vi "FLOW-RATE_read_flow_rate.vi"(4 "error in":errorcluster, 5 "Data t i-1":cluster{"time (s)":dbl, "volume (µl)":dbl}, 6 "FRP out":T1, 7 "Reset":bool) -> (0 "error out":errorcluster, 1 "Data t i":cluster{"time (s)":dbl, "volume (µl)":dbl}, 2 "FR (µl/min)":dbl, 3 "volume (µl)":dbl)   [LabVIEW 2015]
uses:
  <userlib>/Fluigent/Fluigent FRP/FluigentFRP.llb/_frpEnum.ctl
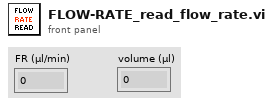
[diagram p1: front panel]
types:
  T1 = typedef "_frpRefNum" = refnum<k1>
  T2 = enum16{"Always On", "Always Off", "Off While Running"}
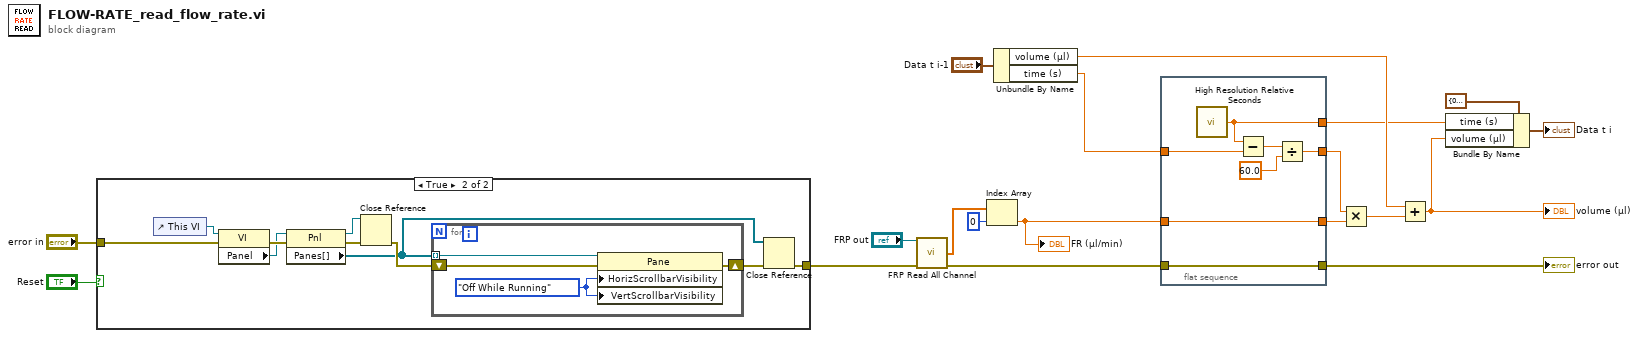
[diagram p0: block diagram]
diagram:
  n1 = case shown="True" "Reset" {
    tunnel: "error in" -> [w20 w22]
    tunnel: [w20 w21] -> w14
    frame False {
    }
    frame True {
      n2 = control-ref of="This VI"() -> (w23:refnum<vi>)
      n3 = property class="VI"(reference=w23, error in=w22) -> (error out=w25:errorcluster, "Panel"=w24:refnum<vi>)  [unwired: 1 out]
      n4 = property class="Pnl"(reference=w24, error in=w25) -> (reference out=w26:refnum<vi>, error out=w27:errorcluster, "Panes[]"=w29:refnum<vi>[])
      n5 = Close Reference(reference=w26, error in (no error)=w27) -> (error out=w30:errorcluster)
      n6 = for {
        tunnel: w29 -> [w34] mode=indexing
        shift-right: [w32] -> w28
        shift-left: w30 -> [w31]
        w33 = T2."Off While Running" ("Horizontal Scrollbar Visibility")
        n7 = property class="Pane"(reference=w34, error in=w31, "HorizScrollbarVisibility"=w33, "VertScrollbarVisibility"=w33) -> (error out=w32:errorcluster)  [unwired: 1 out]
      }
      n8 = Close Reference(reference=w29, error in (no error)=w28) -> (error out=w21:errorcluster)
    }
  }
  n9 = call <userlib>:"FRP Read All Channel.vi"("FRP"="FRP out", "error in (no error)"=w14) -> ("All Flow-Rates"=w16:dbl[], "error out"=w13:errorcluster)  [unwired: 11 in, 1 out]
  n10 = Index Array(array=w16, index=0) -> (element=w12:dbl)
  "FR (µl/min)" <- w12
  n11 = Unbundle By Name("Data t i-1") -> ("volume (µl)"=w5:dbl, "time (s)"=w7:dbl)
  n12 = flat-sequence {
    tunnel: w13 -> [w41]
    tunnel: [w41] -> w9
    tunnel: [w40] -> w3
    tunnel: [w37] -> w10
    tunnel: w12 -> [w36]
    tunnel: [w36] -> w11
    tunnel: w7 -> [w35]
    frame #0 {
      n13 = call <vilib>:"High Resolution Relative Seconds.vi"() -> ("relative seconds"=w40:dbl)
      n14 = Subtract(x=w40, y=w35) -> (x-y=w39:dbl)
      n15 = Divide(x=w39, y=60.0) -> (x/y=w37:dbl)
    }
  }
  n16 = Multiply(x=w10, y=w11) -> (x*y=w6:dbl)
  n17 = Add(x=w5, y=w6) -> (x+y=w1:dbl)
  "volume (µl)" <- w1
  n18 = Bundle By Name(cluster=cluster{"time (s)":dbl, "volume (µl)":dbl} {"time (s)"=0.0, "volume (µl)"=0.0}, "time (s)"=w3, "volume (µl)"=w1) -> (→"Data t i":cluster{"time (s)":dbl, "volume (µl)":dbl})
  "error out" <- w9
